vi "Acquire.vi"(8 "error in":errorcluster, 11 "4081 in":refnum<class "4081.lvclass">) -> (0 "error out":errorcluster, 2 "Acquired":waveform(dbl)[](array[waveform]), 3 "4081 out":refnum<class "4081.lvclass">)   [LabVIEW 2019, in "4081.lvlib" / "4081.lvclass"]
uses:
  Library/4081.lvclass
  C:/Users/Public/Documents/Development/builds/Instruments/Multimeter.lvlibp/Library/Multimeter.lvclass
  C:/Users/Public/Documents/Development/builds/Instruments/Instruments.lvlibp/Library/Instruments.lvclass
  builds/Instruments/Multimeter.lvlibp/Custom Controls/Mode.ctl
  Library/4081.lvclass/4081.ctl
  Accessors/Read Local Resource.vi
  builds/Instruments/Instruments.lvlibp/Accessors/Read dt.vi
  builds/Instruments/Multimeter.lvlibp/Library/Multimeter.lvclass
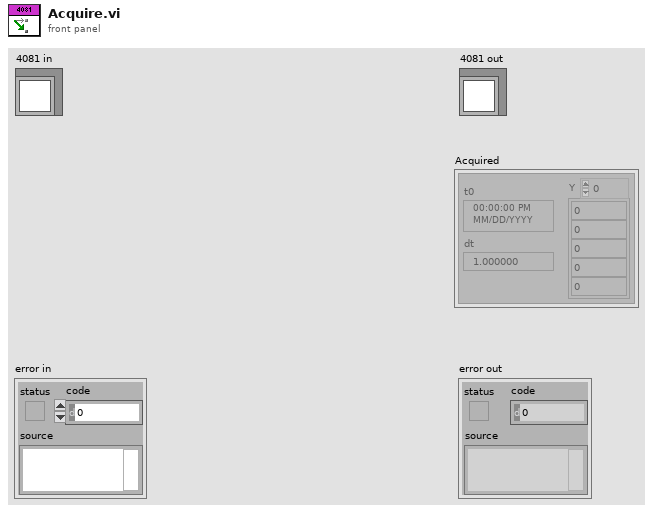
[diagram p1: front panel]
types:
  T1 = typedef "Multimeter.lvlibp/Multimeter.lvclass/Mode.ctl" = enum16{"DC_Volts", "AC_Volts", "DC_Current", "AC_Current", "Resistance_2_Wire", "Resistance_4_Wire", "Diode", "Frequency", "Period", "AC_Volts_DC_Coupled", "Capacitance", "Inductance", "Temperature"}
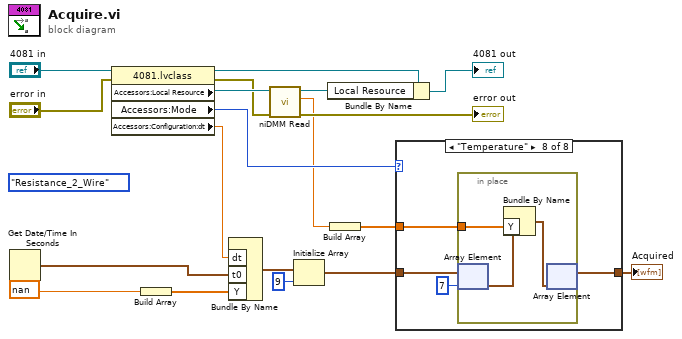
[diagram p0: block diagram]
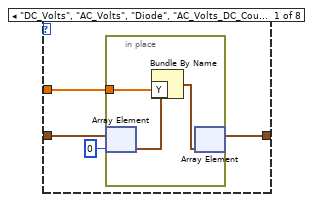
[diagram p2: hidden frame]
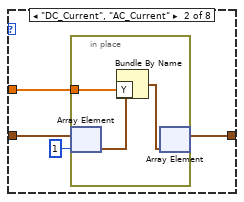
[diagram p3: hidden frame]
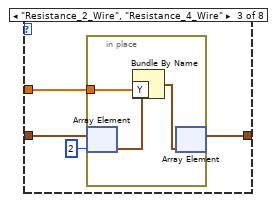
[diagram p4: hidden frame]
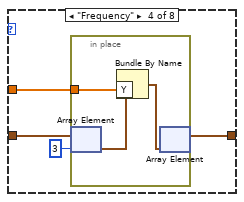
[diagram p5: hidden frame]
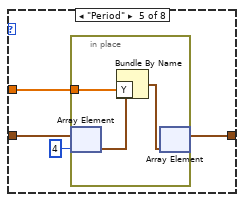
[diagram p6: hidden frame]
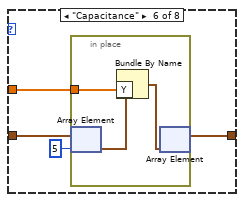
[diagram p7: hidden frame]
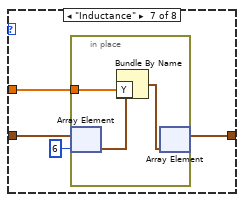
[diagram p8: hidden frame]
diagram:
  (unwired) Mode."Resistance_2_Wire" ("Mode")
  n1 = Get Date/Time In Seconds() -> (seconds since 1Jan1904=w12:timestamp)
  n2 = property class="4081.lvclass"(reference="4081 in", error in="error in") -> (reference out=w15:refnum<class "4081.lvclass">, error out=w13:errorcluster, "Accessors:Local Resource"=w16:refnum<k15>, "Accessors:Mode"=w5:T1, "Accessors:Configuration:dt"=w11:dbl)
  n3 = Build Array(nan) -> (w9:dbl[])
  n4 = Bundle By Name("dt"=w11, "t0"=w12, "Y"=w9) -> (w8:waveform(dbl))  [unwired: 1 in]
  n5 = call <instrlib>:"niDMM Read.vi"("error in (no error)"=w13, "instrument handle"=w16) -> ("error out"=→"error out":errorcluster, "Measurement"=w3:dbl, "instrument handle out"=w18:refnum<k15>)  [unwired: 7 in]
  n6 = Initialize Array(w8, 9 ("dimension size")) -> (w4:waveform(dbl)[])
  n7 = Bundle By Name(cluster=w15, "Local Resource"=w18) -> (→"4081 out":refnum<class "4081.lvclass">)
  n8 = Build Array(w3) -> (w2:dbl[])
  n9 = case shown="\"Temperature\"" w5 {
    tunnel: w4 -> [w23 w30 w37 w44 w51 w58 w65 w72]
    tunnel: [w22 w29 w36 w43 w50 w57 w64 w71] -> w1
    tunnel: w2 -> [w20 w27 w34 w41 w48 w55 w62 w69]
    frame "DC_Volts", "AC_Volts", "Diode", "AC_Volts_DC_Coupled" {
      n10 = in-place {
        in-place-border: w20 -> [w24]
        n11 = in-place-array #1(w23, 0) -> (w26:waveform(dbl))
        n12 = Bundle By Name(cluster=w26, "Y"=w24) -> (w25:waveform(dbl))
        n13 = in-place-array #1(w25) -> (w22:waveform(dbl)[])  [unwired: 1 out]
      }
    }
    frame "DC_Current", "AC_Current" {
      n14 = in-place {
        in-place-border: w27 -> [w31]
        n15 = in-place-array #2(w30, 1) -> (w33:waveform(dbl))
        n16 = Bundle By Name(cluster=w33, "Y"=w31) -> (w32:waveform(dbl))
        n17 = in-place-array #2(w32) -> (w29:waveform(dbl)[])  [unwired: 1 out]
      }
    }
    frame "Resistance_2_Wire", "Resistance_4_Wire" {
      n18 = in-place {
        in-place-border: w34 -> [w38]
        n19 = in-place-array #3(w37, 2) -> (w40:waveform(dbl))
        n20 = Bundle By Name(cluster=w40, "Y"=w38) -> (w39:waveform(dbl))
        n21 = in-place-array #3(w39) -> (w36:waveform(dbl)[])  [unwired: 1 out]
      }
    }
    frame "Frequency" {
      n22 = in-place {
        in-place-border: w41 -> [w45]
        n23 = in-place-array #4(w44, 3) -> (w47:waveform(dbl))
        n24 = Bundle By Name(cluster=w47, "Y"=w45) -> (w46:waveform(dbl))
        n25 = in-place-array #4(w46) -> (w43:waveform(dbl)[])  [unwired: 1 out]
      }
    }
    frame "Period" {
      n26 = in-place {
        in-place-border: w48 -> [w52]
        n27 = in-place-array #5(w51, 4) -> (w54:waveform(dbl))
        n28 = Bundle By Name(cluster=w54, "Y"=w52) -> (w53:waveform(dbl))
        n29 = in-place-array #5(w53) -> (w50:waveform(dbl)[])  [unwired: 1 out]
      }
    }
    frame "Capacitance" {
      n30 = in-place {
        in-place-border: w55 -> [w59]
        n31 = in-place-array #6(w58, 5) -> (w61:waveform(dbl))
        n32 = Bundle By Name(cluster=w61, "Y"=w59) -> (w60:waveform(dbl))
        n33 = in-place-array #6(w60) -> (w57:waveform(dbl)[])  [unwired: 1 out]
      }
    }
    frame "Inductance" {
      n34 = in-place {
        in-place-border: w62 -> [w66]
        n35 = in-place-array #7(w65, 6) -> (w68:waveform(dbl))
        n36 = Bundle By Name(cluster=w68, "Y"=w66) -> (w67:waveform(dbl))
        n37 = in-place-array #7(w67) -> (w64:waveform(dbl)[])  [unwired: 1 out]
      }
    }
    frame "Temperature" {
      n38 = in-place {
        in-place-border: w69 -> [w73]
        n39 = in-place-array #8(w72, 7) -> (w75:waveform(dbl))
        n40 = Bundle By Name(cluster=w75, "Y"=w73) -> (w74:waveform(dbl))
        n41 = in-place-array #8(w74) -> (w71:waveform(dbl)[])  [unwired: 1 out]
      }
    }
  }
  "Acquired" <- w1
